vi "AP2_PDS_aquisition.vi"() -> ()   [LabVIEW 2023]
panel:
  in  "Tab Control 2":enum32{"Image Acquistion Settings"}(tab)
  in  "Threshold range":cluster{"Lower value":sgl, "Upper value":sgl}={"Lower value"=6.0, "Upper value"=1024.0}
  in  "Region of interest":i32[](array[numeric])=[0, 0, 1020, 1020]
  in  "Number of buffers":u32=100
  in  "Frame timeout (ms)":u32=1000
  in  "Tab Control":T1(tab)
  in  "Scan Step Size / nm":dbl=1.0
  in  "Scan Start / nm":dbl=540.0
  in  "Scan End / nm":dbl=550.0
  in  "Number of Frames Per Wavelength":i32=700
  in  "Scan button":bool
  in  "Cancel Scan Button":bool
  out "Scan In Progress?":bool
  out "FPS":dbl=52.63157894736842
  out "RT Pulse Energy / J":dbl=0.00298
  out "Current Laser Position / nm":dbl=0.00298
  in  "Frequency Doubling":bool
  in  "PDS Display Tabs":enum32{"Raw PDS", "Power Scaled PDS"}(tab)
  out "RT Raw PDS":cluster{dbl[], dbl[]}(graph)
  out "RT Scaled PDS":cluster{dbl[], dbl[]}(graph)
  in  "Stop":bool
  # "AP-2 PDS Acquisition"
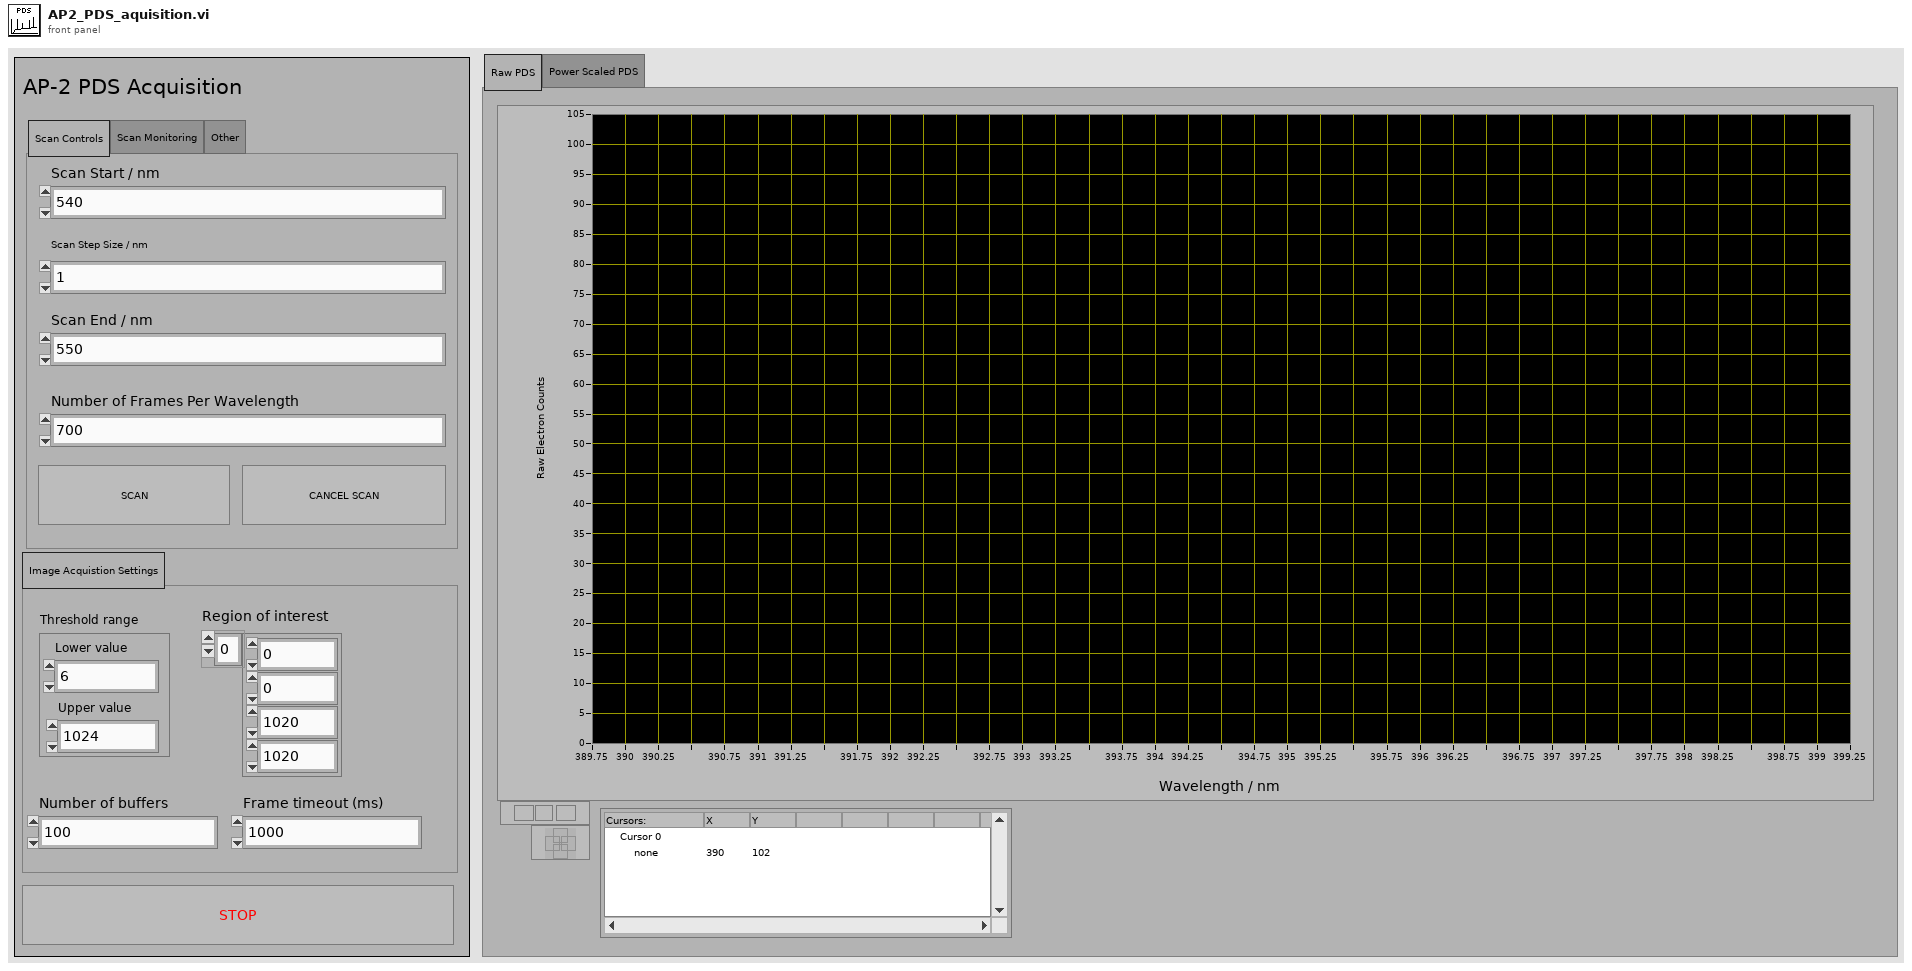
[diagram p1: front panel]
types:
  T1 = enum32{"Scan Controls", "Scan Monitoring", "Other"}
  T2 = cluster{"Raw PDS Data":cluster{dbl[], dbl[]}, "Power Scaled PDS Data":cluster{dbl[], dbl[]}}
  T3 = cluster{"Region of interest":i32[], "Number of buffers":u32, "Frame timeout (ms)":u32}
  T4 = cluster{"queue out":refnum<queue>, "error out":errorcluster}
  T5 = cluster{"OphirLMMeasurementLib.ICoLMMeasurement2":refnum<k7>, "Error":errorcluster, "hDevice":i32}
  T6 = cluster{"notifier out":refnum<notifier>, "error out":errorcluster}
  T7 = cluster{"Cancel Scan Notifier":cluster{"notifier out":refnum<notifier>, "error out":errorcluster}, "Laser Power Q":cluster{"queue out":refnum<queue>, "error out":errorcluster}, "Electron Count Q":cluster{"queue out":refnum<queue>, "error out":errorcluster}}
  T8 = cluster{"Upper bound":dbl, "Step Size":dbl, "Lower Bound":dbl}
  T9 = cluster{"Aquistion Frame Number":i32, "Laser Parameters":cluster{"Upper bound":dbl, "Step Size":dbl, "Lower Bound":dbl}}
  T10 = cluster{"Tuning Spline Path":path, "Frequency Doubling":bool}
  T11 = cluster{"Power Reading ":dbl, "T imestamp":dbl, "Status":i32}
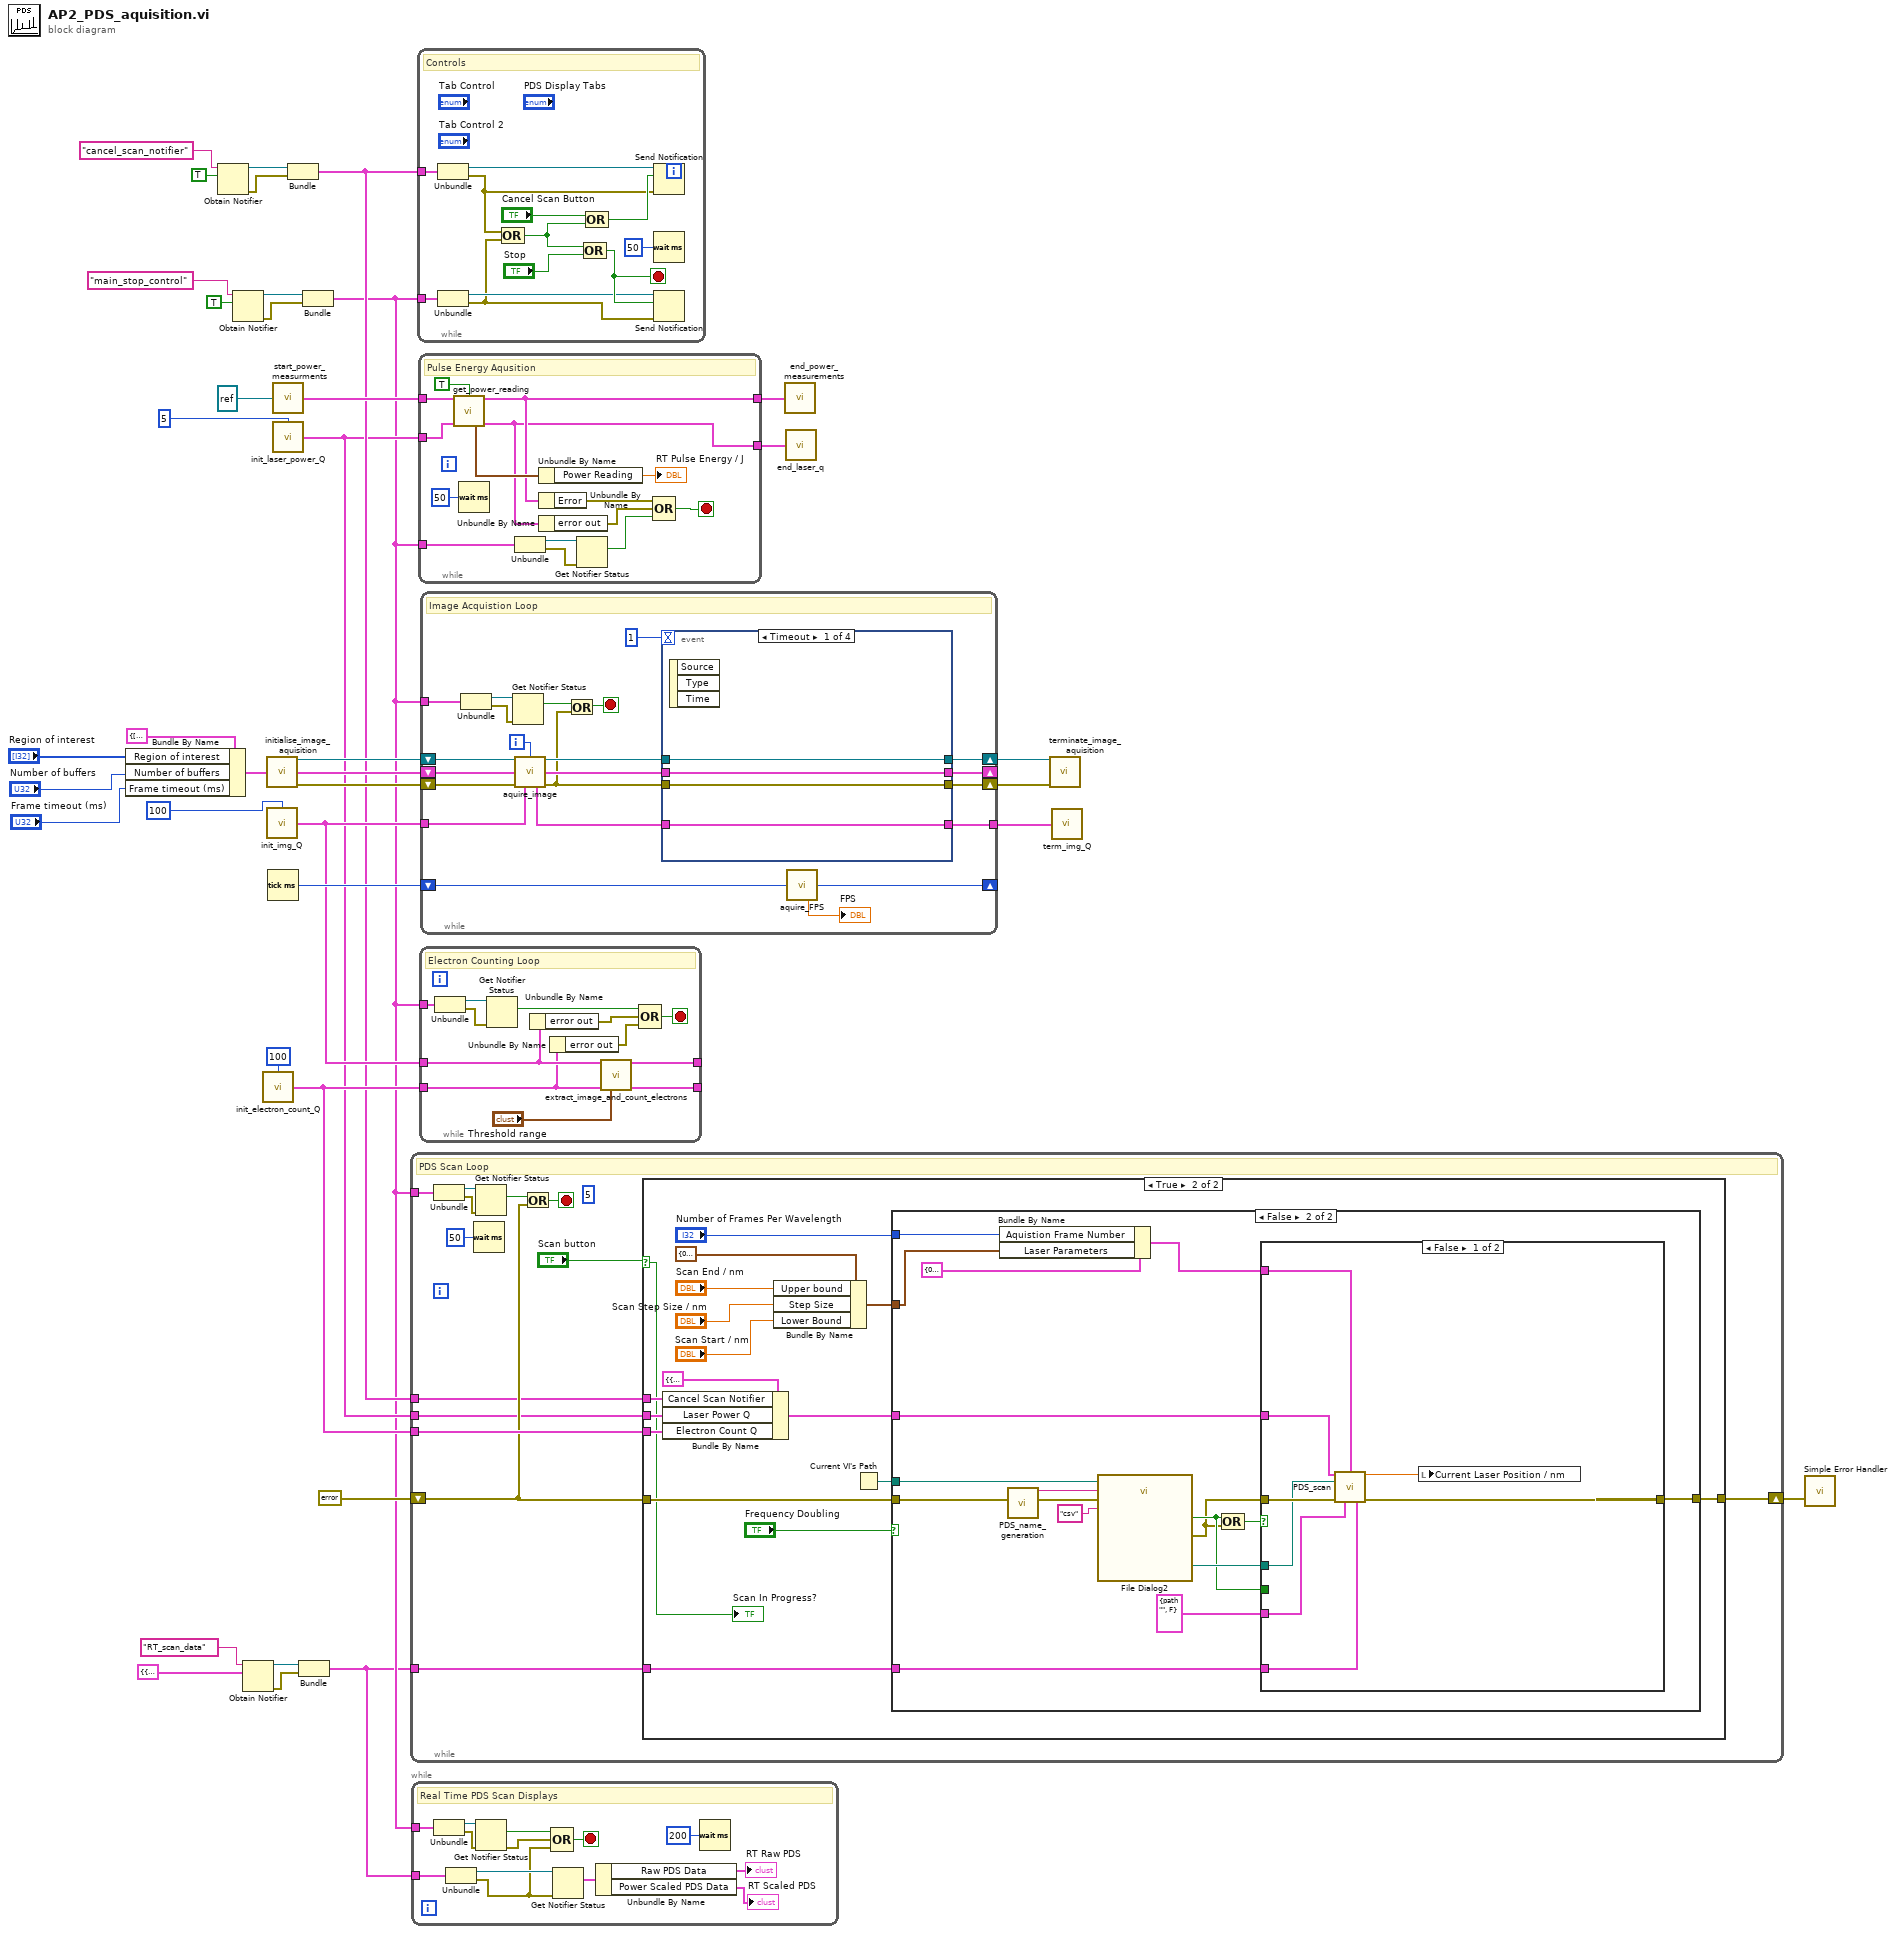
[diagram p0: block diagram]
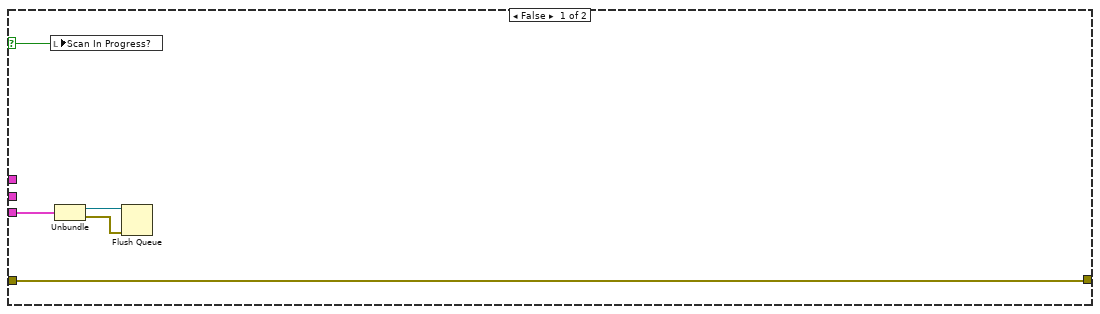
[diagram p2: hidden frame]
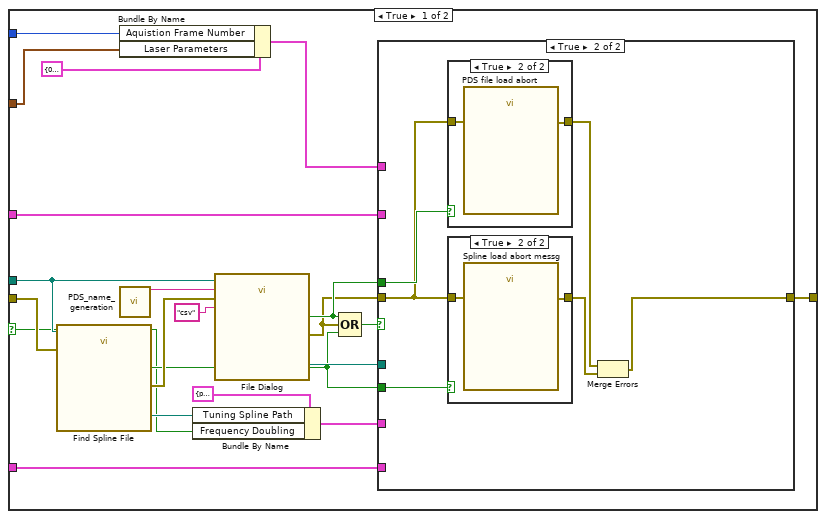
[diagram p3: hidden frame]
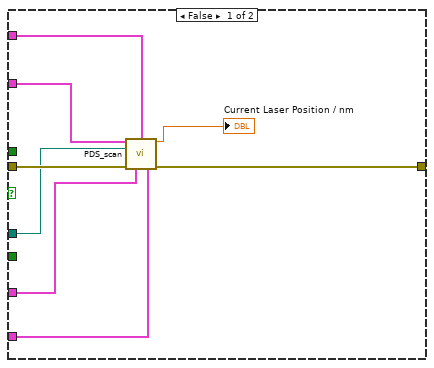
[diagram p4: hidden frame]
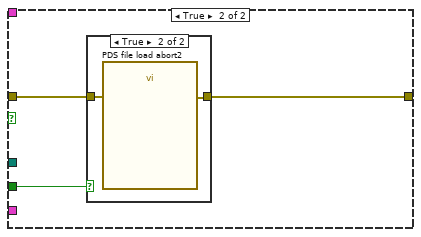
[diagram p7: hidden frame]
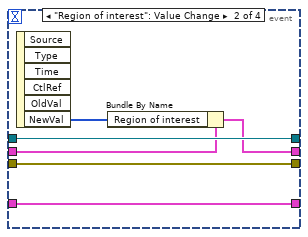
[diagram p9: hidden frame]
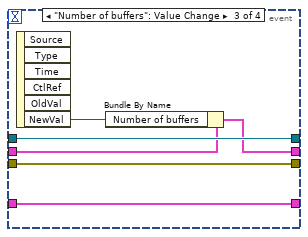
[diagram p10: hidden frame]
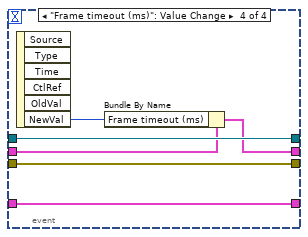
[diagram p11: hidden frame]
diagram:
  n1 = Bundle By Name(cluster=T3 {"Region of interest"=[], "Number of buffers"=0, "Frame timeout (ms)"=1000}, "Region of interest"="Region of interest", "Number of buffers"="Number of buffers", "Frame timeout (ms)"="Frame timeout (ms)") -> (w33:T3)
  n2 = Obtain Notifier(name (unnamed)="cancel_scan_notifier", notification data type=TRUE) -> (notifier out=w13:refnum<notifier>, error out=w12:errorcluster)  [unwired: 2 in, 1 out]
  n3 = Obtain Notifier(name (unnamed)="main_stop_control", notification data type=TRUE) -> (notifier out=w16:refnum<notifier>, error out=w15:errorcluster)  [unwired: 2 in, 1 out]
  n4 = Obtain Notifier(name (unnamed)="RT_scan_data", notification data type=T2 {"Raw PDS Data"={[389.999964, 391.000163, 391.99987, 392.999885, 394.000206, 395.00003999999996, 396.000181, 396.99983699999996, 398.00019599999996, 399.000071, 399.99985999999996], [2.0, 0.0, 0.0, 0.0, 0.0, 0.0, 0.0, 0.0, 0.0, 0.0, 0.0]}, "Power Scaled PDS Data"={[389.999964, 391.000163, 391.99987, 392.999885, 394.000206, 395.00003999999996, 396.000181, 396.99983699999996, 398.00019599999996, 399.000071, 399.99985999999996], [inf, nan, nan, nan, nan, nan, nan, nan, nan, nan, nan]}} ("RT PDS Data Sets")) -> (notifier out=w4:refnum<notifier>, error out=w3:errorcluster)  [unwired: 2 in, 1 out]
  n5 = call "init_electron_count_Q.vi"("max queue size (-1, unlimited)"=100) -> ("Electron Count Q Out"=w21:T4)  [unwired: 14 in]
  n6 = call "initialise_image_aquisition.vi"("Imaging Variables In"=w33) -> ("IMAQ Session Out"=w36:refnum<k11>, "Imaging Variables Out"=w32:T3, "error out"=w35:errorcluster)  [unwired: 11 in, 1 out]
  n7 = call "init_img_Q.vi"("max queue size (-1, unlimited)"=100) -> ("Image Q Out"=w27:T4)  [unwired: 14 in]
  n8 = Tick Count (ms)() -> (millisecond timer value=w28:u32)
  n9 = call "start_power_measurments.vi"("OphirLMMeasurementLib.ICoLMMeasurement2"=refnum<k7> refnum) -> ("Power Meter Connection Data Out"=w39:T5)  [unwired: 14 in]
  n10 = call "init_laser_power_Q.vi"("max queue size (-1, unlimited)"=5) -> ("Laser Power Q"=w8:T4)  [unwired: 14 in]
  n11 = Bundle("notifier out"=w13, "error out"=w12) -> (w10:T6)  [unwired: 1 in]
  n12 = Bundle("notifier out"=w4, "error out"=w3) -> (w1:T6)  [unwired: 1 in]
  n13 = Bundle("notifier out"=w16, "error out"=w15) -> (w2:T6)  [unwired: 1 in]
  n14 = while {
    shift-right: [w52] -> w22
    shift-left: errorcluster {"status"=FALSE, "code"=0, "source"=""} ("error out") -> [w49]
    tunnel: w21 -> [w51]
    tunnel: w2 -> [w47]
    tunnel: w10 -> [w44]
    tunnel: w8 -> [w42]
    tunnel: w1 -> [w40]
    stop <- w48 stop-if-true
    (unwired) 5
    # "PDS Scan Loop"
    n15 = Unbundle(w47) -> ("notifier out"=w46:refnum<notifier>, "error out"=w45:errorcluster)
    n16 = Wait (ms)(milliseconds to wait=u32 50) -> ()  [unwired: 1 out]
    n17 = Get Notifier Status(notifier=w46, error in (no error)=w45) -> (current notification=w50:bool)  [unwired: 4 out]
    n18 = Or(x=w50, y=w49) -> (x .or. y?=w48:bool)
    n19 = case shown="True" "Scan button" {
      selector: "Scan button" -> [w53 w58]
      tunnel: [w57 w74] -> w52
      tunnel: w51 -> [w56 w73]
      tunnel: w49 -> [w57 w72]
      tunnel: w44 -> [_ w71]
      tunnel: w42 -> [_ w70]
      tunnel: w40 -> [_ w59]
      frame False {
        n20 = local write "Scan In Progress?"(w53) -> ()
        n21 = Unbundle(w56) -> ("queue out"=w55:refnum<queue>, "error out"=w54:errorcluster)
        n22 = Flush Queue(queue=w55, error in (no error)=w54) -> ()  [unwired: 3 out]
      }
      frame True {
        n23 = Bundle By Name(cluster=T7 {"Cancel Scan Notifier"={"notifier out"=refnum, "error out"={"status"=FALSE, "code"=0, "source"=""}}, "Laser Power Q"={"queue out"=refnum, "error out"={"status"=FALSE, "code"=0, "source"=""}}, "Electron Count Q"={"queue out"=refnum, "error out"={"status"=FALSE, "code"=0, "source"=""}}}, "Cancel Scan Notifier"=w71, "Laser Power Q"=w70, "Electron Count Q"=w73) -> (w61:T7)
        n24 = Bundle By Name(cluster=T8 {"Upper bound"=0.0, "Step Size"=0.0, "Lower Bound"=0.0}, "Upper bound"="Scan End / nm", "Step Size"="Scan Step Size / nm", "Lower Bound"="Scan Start / nm") -> (w65:T8)
        n25 = Current VI's Path() -> (path=w63:path)
        n26 = case shown="False" "Frequency Doubling" {
          selector: "Frequency Doubling" -> [w81 _]
          tunnel: w65 -> [w78 w120]
          tunnel: "Number of Frames Per Wavelength" -> [w79 w121]
          tunnel: w63 -> [w91 w123]
          tunnel: w72 -> [w95 w124]
          tunnel: [w85 w125] -> w74
          tunnel: w61 -> [w76 w118]
          tunnel: w59 -> [w75 w116]
          frame True {
            n27 = call "Find Spline File"("start path"=w91, "error in"=w95) -> ("selected path"=w84:path, "cancelled"=w88:bool, "error out"=w92:errorcluster)  [unwired: 10 in, 1 out]
            n28 = Bundle By Name(cluster=T9 {"Aquistion Frame Number"=0, "Laser Parameters"={"Upper bound"=0.0, "Step Size"=0.0, "Lower Bound"=0.0}}, "Aquistion Frame Number"=w79, "Laser Parameters"=w78) -> (w77:T9)
            n29 = call "PDS_name_generation.vi"() -> ("Generic Name"=w94:string)  [unwired: 15 in]
            n30 = Bundle By Name(cluster=T10 {"Tuning Spline Path"=path "", "Frequency Doubling"=FALSE}, "Tuning Spline Path"=w84, "Frequency Doubling"=w81) -> (w82:T10)
            n31 = call "File Dialog"("start path"=w91, "default name"=w94, "error in"=w92, "pattern (all files)"="csv") -> ("selected path"=w89:path, "cancelled"=w87:bool, "error out"=w86:errorcluster)  [unwired: 8 in, 1 out]
            n32 = Compound Arithmetic op=OR(w87, w86, w88) -> (w90:bool)
            n33 = case shown="True" w90 {
              tunnel: w89 -> [w101 _]
              tunnel: w88 -> [_ w109]
              tunnel: w86 -> [w103 w107]
              tunnel: w87 -> [_ w108]
              tunnel: [w102 w105] -> w85
              tunnel: w82 -> [w98 _]
              tunnel: w77 -> [w100 _]
              tunnel: w76 -> [w99 _]
              tunnel: w75 -> [w96 _]
              frame False {
                n34 = call "PDS_scan.vi"("Q Data In"=w99, "Scan Parameters"=w100, "file path (dialog if empty)"=w101, "error in (no error)"=w103, "Freq Doubling Controls"=w98, "RT Scan Data"=w96) -> ("Current Laser Position / nm"=→"Current Laser Position / nm":dbl, "error out"=w102:errorcluster)  [unwired: 8 in]
              }
              frame True {
                n35 = case shown="True" w108 {
                  tunnel: w107 -> [w110 w112]
                  tunnel: [w110 w111] -> w106
                  frame False {
                  }
                  frame True {
                    n36 = call "PDS file load abort"("error in (no error)"=w112) -> ("error out"=w111:errorcluster)  [unwired: 9 in, 1 out]
                  }
                }
                n37 = case shown="True" w109 {
                  tunnel: w107 -> [w113 w115]
                  tunnel: [w113 w114] -> w104
                  frame False {
                  }
                  frame True {
                    n38 = call "Spline load abort messg"("error in (no error)"=w115) -> ("error out"=w114:errorcluster)  [unwired: 9 in, 1 out]
                  }
                }
                n39 = Merge Errors(w106, w104) -> (w105:errorcluster)
              }
            }
          }
          frame False {
            n40 = Bundle By Name(cluster=T9 {"Aquistion Frame Number"=0, "Laser Parameters"={"Upper bound"=0.0, "Step Size"=0.0, "Lower Bound"=0.0}}, "Aquistion Frame Number"=w121, "Laser Parameters"=w120) -> (w119:T9)
            n41 = call "PDS_name_generation.vi"() -> ("Generic Name"=w131:string)  [unwired: 15 in]
            n42 = call "File Dialog2"("start path"=w123, "default name"=w131, "error in"=w124, "pattern (all files)"="csv") -> ("selected path"=w128:path, "cancelled"=w127:bool, "error out"=w126:errorcluster)  [unwired: 8 in, 1 out]
            n43 = Compound Arithmetic op=OR(w127, w126) -> (w129:bool)
            n44 = case shown="False" w129 {
              tunnel: w128 -> [w137 _]
              tunnel: w126 -> [w139 w141]
              tunnel: w127 -> [_ w142]
              tunnel: [w138 w140] -> w125
              tunnel: w119 -> [w136 _]
              tunnel: w118 -> [w135 _]
              tunnel: T10 {"Tuning Spline Path"=path "", "Frequency Doubling"=FALSE} ("Freq Doubling Controls") -> [w134 _]
              tunnel: w116 -> [w132 _]
              frame False {
                n45 = call "PDS_scan.vi"("Q Data In"=w135, "Scan Parameters"=w136, "file path (dialog if empty)"=w137, "error in (no error)"=w139, "Freq Doubling Controls"=w134, "RT Scan Data"=w132) -> ("Current Laser Position / nm"=w133:dbl, "error out"=w138:errorcluster)  [unwired: 8 in]
                n46 = local write "Current Laser Position / nm"(w133) -> ()
              }
              frame True {
                n47 = case shown="True" w142 {
                  tunnel: w141 -> [w143 w145]
                  tunnel: [w143 w144] -> w140
                  frame False {
                  }
                  frame True {
                    n48 = call "PDS file load abort2"("error in (no error)"=w145) -> ("error out"=w144:errorcluster)  [unwired: 9 in, 1 out]
                  }
                }
              }
            }
          }
        }
        "Scan In Progress?" <- w58
      }
    }
  }
  n49 = while {
    tunnel: w2 -> [w153]
    tunnel: w1 -> [w151]
    stop <- w147 stop-if-true
    # "Real Time PDS Scan Displays"
    n50 = Unbundle(w153) -> ("notifier out"=w155:refnum<notifier>, "error out"=w154:errorcluster)
    n51 = Unbundle(w151) -> ("notifier out"=w152:refnum<notifier>, "error out"=w148:errorcluster)
    n52 = Get Notifier Status(notifier=w155, error in (no error)=w154) -> (current notification=w150:bool, error out=w149:errorcluster)  [unwired: 3 out]
    n53 = Compound Arithmetic op=OR(w150, w149, w148) -> (w147:bool)
    n54 = Get Notifier Status(notifier=w152, error in (no error)=w148) -> (current notification=w158:T2)  [unwired: 4 out]
    n55 = Unbundle By Name(w158) -> ("Raw PDS Data"=→"RT Raw PDS":cluster{dbl[], dbl[]}, "Power Scaled PDS Data"=→"RT Scaled PDS":cluster{dbl[], dbl[]})
    n56 = Wait (ms)(milliseconds to wait=u32 200) -> ()  [unwired: 1 out]
  }
  n57 = while {
    tunnel: w2 -> [w163]
    tunnel: w10 -> [w161]
    stop <- w166 stop-if-true
    # "Controls"
    n58 = Unbundle(w161) -> ("notifier out"=w159:refnum<notifier>, "error out"=w160:errorcluster)
    n59 = Unbundle(w163) -> ("notifier out"=w164:refnum<notifier>, "error out"=w162:errorcluster)
    n60 = Compound Arithmetic op=OR(w160, w162) -> (w169:bool)
    n61 = Compound Arithmetic op=OR(w169, "Stop") -> (w166:bool)
    n62 = Compound Arithmetic op=OR("Cancel Scan Button", w169) -> (w167:bool)
    n63 = Send Notification(notification=w167, notifier=w159, error in (no error)=w160) -> ()  [unwired: 2 out]
    n64 = Wait (ms)(milliseconds to wait=u32 50) -> ()  [unwired: 1 out]
    n65 = Send Notification(notification=w166, notifier=w164, error in (no error)=w162) -> ()  [unwired: 2 out]
  }
  n66 = while {
    tunnel: w39 -> [w185]
    tunnel: w8 -> [w184]
    tunnel: [w180] -> w37
    tunnel: [w179] -> w38
    tunnel: w2 -> [w173]
    stop <- w176 stop-if-true
    # "Pulse Energy Aqusition"
    n67 = call "get_power_reading.vi"("Power Meter Connection Data In"=w185, "Q Laser Data?"=TRUE, "Laser Power Q In"=w184) -> ("Power Meter Connection Data Out"=w180:T5, "Data Out"=w183:T11, "Laser Power Q Out"=w179:T4)  [unwired: 9 in, 1 out]
    n68 = Wait (ms)(milliseconds to wait=u32 50) -> ()  [unwired: 1 out]
    n69 = Unbundle(w173) -> ("notifier out"=w175:refnum<notifier>, "error out"=w174:errorcluster)
    n70 = Unbundle By Name(w183) -> ("Power Reading"=→"RT Pulse Energy / J":dbl)
    n71 = Unbundle By Name(w180) -> ("Error"=w178:errorcluster)
    n72 = Unbundle By Name(w179) -> ("error out"=w177:errorcluster)
    n73 = Get Notifier Status(notifier=w175, error in (no error)=w174) -> (current notification=w172:bool)  [unwired: 4 out]
    n74 = Compound Arithmetic op=OR(w178, w177, w172) -> (w176:bool)
  }
  n75 = while {
    tunnel: w27 -> [w196]
    tunnel: w21 -> [w195]
    tunnel: w2 -> [w189]
    tunnel: [w187] -> _
    tunnel: [w186] -> _
    stop <- w191 stop-if-true
    # "Electron Counting Loop"
    n76 = Unbundle(w189) -> ("notifier out"=w190:refnum<notifier>, "error out"=w188:errorcluster)
    n77 = Get Notifier Status(notifier=w190, error in (no error)=w188) -> (current notification=w194:bool)  [unwired: 4 out]
    n78 = Unbundle By Name(w196) -> ("error out"=w193:errorcluster)
    n79 = Unbundle By Name(w195) -> ("error out"=w192:errorcluster)
    n80 = call "extract_image_and_count_electrons.vi"("Image Q In"=w196, "Electron Count Q In"=w195, "Range"="Threshold range") -> ("Image Q Out"=w187:T4, "Electron Count Q Out"=w186:T4)  [unwired: 10 in, 1 out]
    n81 = Compound Arithmetic op=OR(w194, w193, w192) -> (w191:bool)
  }
  n82 = while {
    shift-right: [w218] -> w30
    shift-left: w36 -> [w215]
    shift-right: [w216] -> w29
    shift-left: w35 -> [w214]
    tunnel: w27 -> [w208]
    tunnel: [w207] -> w31
    shift-right: [w217] -> _
    shift-left: w32 -> [w211]
    shift-right: [w205] -> _
    shift-left: w28 -> [w206]
    tunnel: w2 -> [w198]
    i -> [w213]
    stop <- w203 stop-if-true
    # "Image Acquistion Loop"
    n83 = Unbundle(w198) -> ("notifier out"=w200:refnum<notifier>, "error out"=w199:errorcluster)
    n84 = Get Notifier Status(notifier=w200, error in (no error)=w199) -> (current notification=w202:bool)  [unwired: 4 out]
    n85 = call "aquire_image.vi"("IMAQ Session In"=w215, "Buffer to extract"=w213, "Imaging Variables In"=w211, "error in (no error)"=w214, "Img Q Data In"=w208) -> ("IMAQ Session Out"=w212:refnum<k11>, "Imaging Variables Out"=w210:T3, "Img Q Data Out"=w209:T4, "error out"=w201:errorcluster)  [unwired: 7 in]
    n86 = Or(x=w202, y=w201) -> (x .or. y?=w203:bool)
    n87 = event shown="[0] Timeout" {
      selector: _ -> [_ _ _ _]
      dyn-events: _ -> [_ _ _ _]
      timeout: 1 -> [_ _ _ _]
      tunnel: w212 -> [w223 w229 w235 w241]
      tunnel: w201 -> [w222 w228 w234 w240]
      tunnel: [w223 w229 w235 w241] -> w218
      tunnel: [w222 w228 w234 w240] -> w216
      tunnel: w210 -> [w221 w226 w232 w238]
      tunnel: [w221 w225 w231 w237] -> w217
      tunnel: w209 -> [w220 w227 w233 w239]
      tunnel: [w220 w227 w233 w239] -> w207
      event Timeout {
        n88 = event-data() -> ()  [unwired: 1 in, 3 out]
      }
      event "Region of interest": Value Change {
        n89 = event-data() -> ("NewVal"=w224:i32[])  [unwired: 1 in, 5 out]
        n90 = Bundle By Name(cluster=w226, "Region of interest"=w224) -> (w225:T3)
      }
      event "Number of buffers": Value Change {
        n91 = event-data() -> ("NewVal"=w230:u32)  [unwired: 1 in, 5 out]
        n92 = Bundle By Name(cluster=w232, "Number of buffers"=w230) -> (w231:T3)
      }
      event "Frame timeout (ms)": Value Change {
        n93 = event-data() -> ("NewVal"=w236:u32)  [unwired: 1 in, 5 out]
        n94 = Bundle By Name(cluster=w238, "Frame timeout (ms)"=w236) -> (w237:T3)
      }
    }
    n95 = call "aquire_FPS.vi"("Time Value In /ms"=w206) -> ("Time Value Out /ms"=w205:u32, "FPS"=→"FPS":dbl)  [unwired: 12 in, 1 out]
  }
  n96 = call "end_power_measurements.vi"("Power Meter Connection Data In"=w37) -> ()  [unwired: 14 in, 1 out]
  n97 = call "end_laser_q.vi"("Laser Power Q In"=w38) -> ()  [unwired: 14 in, 1 out]
  n98 = call "terminate_image_aquisition.vi"("IMAQ Session In"=w30, "error in (no error)"=w29) -> ()  [unwired: 13 in, 1 out]
  n99 = call "term_img_Q.vi"("Image Q Out"=w31) -> ()  [unwired: 14 in, 1 out]
  n100 = call <vilib>:"Simple Error Handler.vi"("error in (no error)"=w22) -> ()  [unwired: 4 in, 5 out]
